vi "Conv_Killograms_Pounds.vi"(10 "Pounds":dbl) -> (2 "Killograms":dbl)   [LabVIEW 2019, in "Trajectory_Library.lvlib"]
doc: "Convert mass in kilograms to pounds.\n\nInput:\n - kilograms -- mass in kilograms\n\nOutputs:\n - pounds -- mass in pounds"
uses:
  Trajectory_Library.lvlib
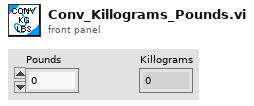
[diagram p1: front panel]
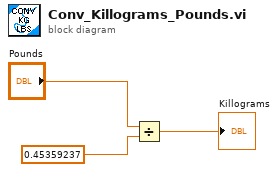
[diagram p0: block diagram]
diagram:
  n1 = Divide(x="Pounds", y=0.45359237) -> (x/y=→"Killograms":dbl)
